vi "solar_tcp Read.vi"(6 "Suppress Errors? (T)":bool=TRUE, 8 "error in (no error)":errorcluster, 9 "Read Timeout (0ms)":i32, 11 "TCP Data in":T1={"Connected"=FALSE, "Config"={"TCPServer"=enum."SERVER", "ServerPort"=0, "IPAddress"="", "ClientPort"=0, "HdrSizeBytes"=4, "HdrLenSubtractBytes"=0, "HdrLenOffsetBits"=0, "HdrLenSizeBits"=32}, "Clients"=[], "ConnectionID"=refnum, "Debug"=[]} {"Debug"."Time" format="%<%Y-%m-%d\n%H:%M:%S%3u>T"}) -> (0 "error out":errorcluster, 1 "Connected":bool, 2 "Message Read":string, 3 "TCP Data out":T1 {"Debug"."Time" format="%<%Y-%m-%d\n%H:%M:%S%3u>T"})   [LabVIEW 2018]
doc: "This reads a message on the TCP connection. Set <b>Read Timeout</b> to wait for incoming message."
uses:
  solar_tcp_ctl Action.ctl
  solar_tcp_ctl Data.ctl
  solar_tcp_ctl Config.ctl
  solar_tcp_ctl Debug.ctl
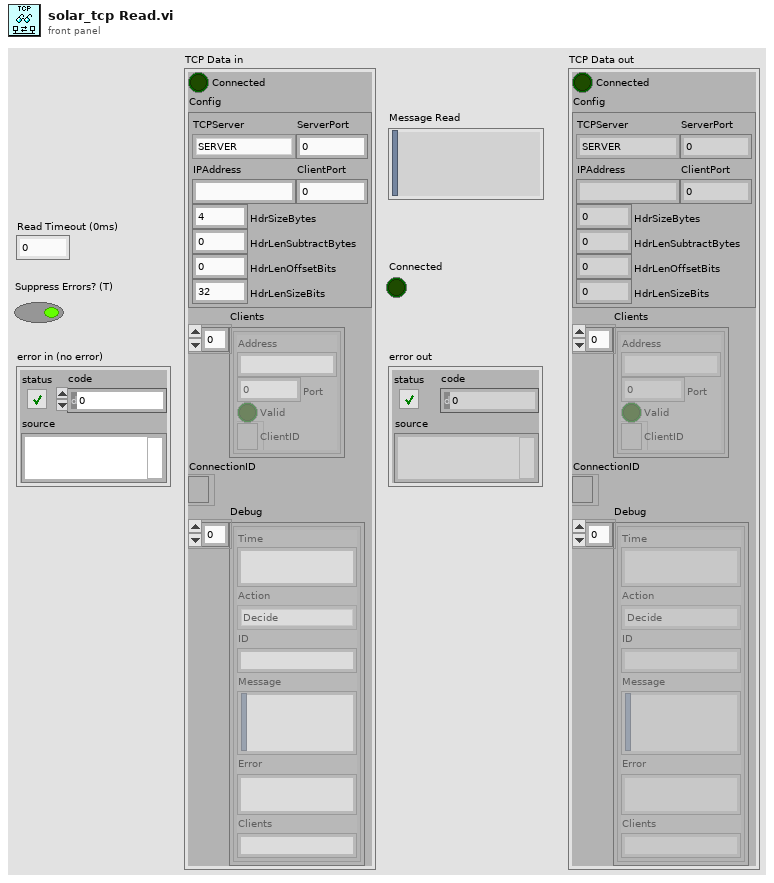
[diagram p1: front panel]
types:
  T1 = typedef "solar_tcp_ctl Data.ctl" = cluster{"Connected":bool, "Config":T2, "Clients":cluster{"Address":string, "Port":u16, "Valid":bool, "ClientID":refnum<k5>}[], "ConnectionID":refnum<k5>, "Debug":T3[]}
  T2 = typedef "solar_tcp_ctl Config.ctl" = cluster{"TCPServer":enum8{"SERVER", "CLIENT"}, "ServerPort":u16, "IPAddress":string, "ClientPort":u16, "HdrSizeBytes":i32, "HdrLenSubtractBytes":i32, "HdrLenOffsetBits":i32, "HdrLenSizeBits":i32}
  T3 = typedef "solar_tcp_ctl Debug.ctl" = cluster{"Time":timestamp, "Action":T4, "ID":string, "Message":string, "Error":string, "Clients":string}
  T4 = typedef "solar_tcp_ctl Action.ctl" = enum16{"Decide", "CreateListener", "Open", "Read", "Write", "Close", "Shutdown", "Done", "ChangePort"}
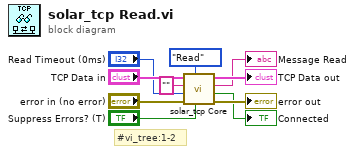
[diagram p0: block diagram]
diagram:
  # "#vi_tree:1-2"
  n1 = call "solar_tcp Core.vi"("Suppress Errors? (T)"="Suppress Errors? (T)", "Action"=solar_tcp_ctl_Action."Read", "error in (no error)"="error in (no error)", "Read Timeout (0ms)"="Read Timeout (0ms)", "Message to Send"="", "TCP Data in"="TCP Data in") -> ("error out"=→"error out":errorcluster, "Connected"=→"Connected":bool, "Message Read/Sent"=→"Message Read":string, "TCP Data out"=→"TCP Data out":T1)  [unwired: 2 in]
